vi "ReadData.vi"(8 "error in (no error)":errorcluster, 11 "object in":refnum<class "RS232.lvclass">) -> (0 "error out":errorcluster, 2 "read buffer":string, 3 "object out":refnum<class "RS232.lvclass">)   [LabVIEW 2019, in "RS232.lvclass"]
uses:
  RS232.lvclass
  RS232.lvclass/RS232.ctl
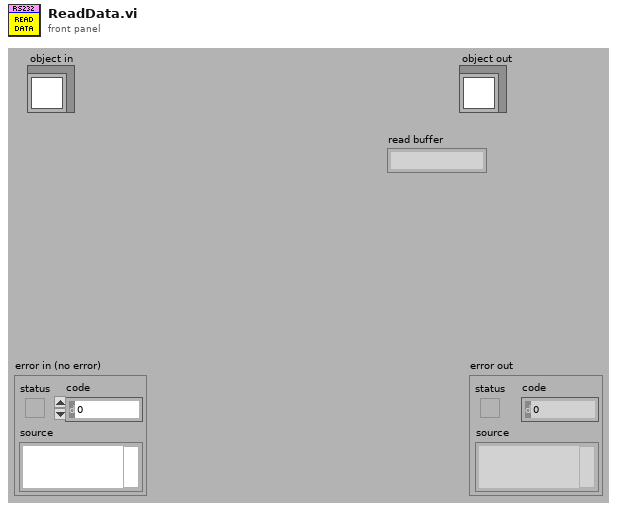
[diagram p1: front panel]
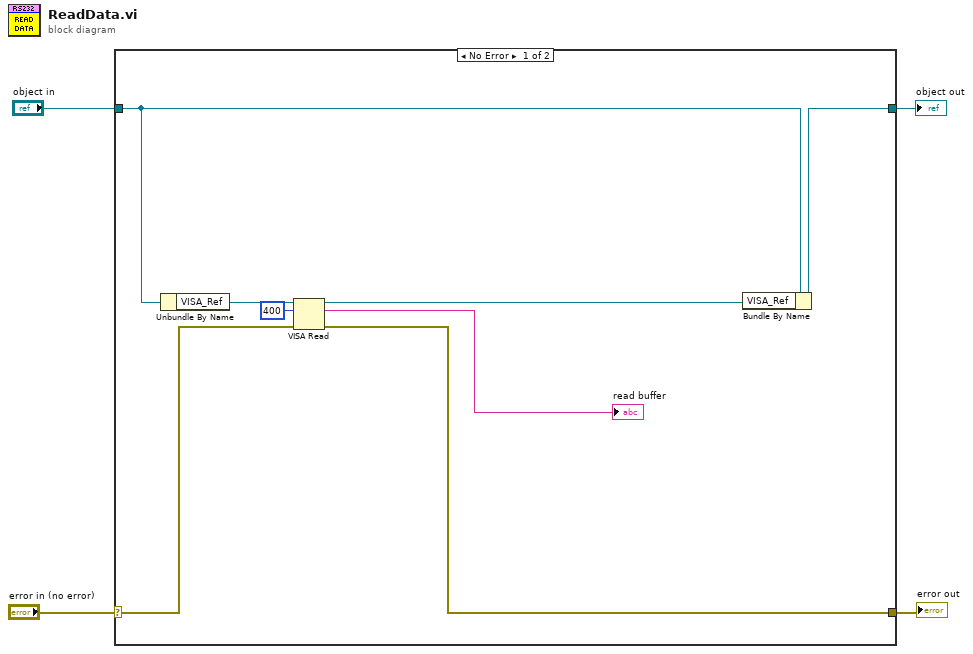
[diagram p0: block diagram]
diagram:
  n1 = case shown="No Error" "error in (no error)" {
    selector: "error in (no error)" -> [w9 w14]
    tunnel: [w8 w14] -> w3
    tunnel: [w7 w13] -> w1
    tunnel: "object in" -> [w12 w13]
    frame No Error {
      n2 = Unbundle By Name(w12) -> ("VISA_Ref"=w11:refnum<visa-resource-name>)
      n3 = VISA Read(VISA resource name=w11, byte count=u32 400, error in (no error)=w9) -> (VISA resource name out=w6:refnum<visa-resource-name>, read buffer=→"read buffer":string, error out=w8:errorcluster)  [unwired: 1 out]
      n4 = Bundle By Name(cluster=w12, "VISA_Ref"=w6) -> (w7:refnum<class "RS232.lvclass">)
    }
    frame Error {
    }
  }
  "error out" <- w3
  "object out" <- w1
